vi "Calculation for heating four glasses.vi"(0 "Заданная температура":dbl[](array[numeric]), 1 "Текущая температура":dbl[](array[numeric]), 2 "Прошлая температура":dbl[](array[numeric]), 3 "Суммарная (прошлая) температура":dbl[](array[numeric]), 4 "Время прошлое":dbl[](array[numeric]), 5 "Время настоящее":dbl[](array[numeric])) -> (14 "Время во включенном состоянии":dbl[](array[numeric]), 19 "Суммарная температура":dbl[](array[numeric]))   [LabVIEW 2016]
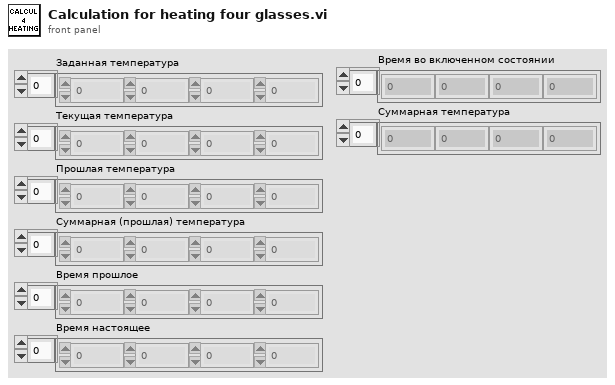
[diagram p1: front panel]
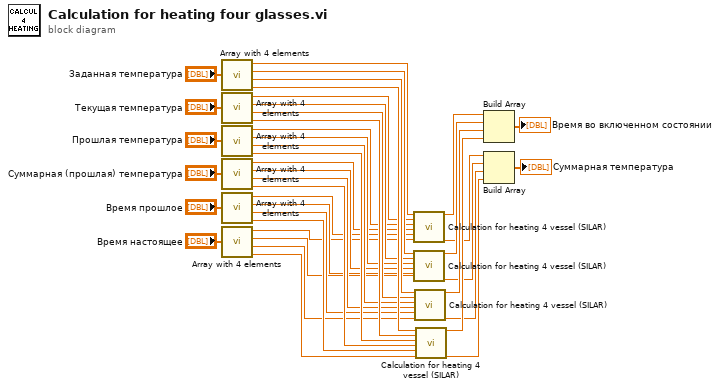
[diagram p0: block diagram]
diagram:
  n1 = call "Array with 4 elements.vi"("Array with 4 elements"="Заданная температура") -> ("element 3"=w35:dbl, "element 2"=w36:dbl, "element 1"=w38:dbl, "element 0"=w39:dbl)  [unwired: 7 in]
  n2 = call "Array with 4 elements.vi"("Array with 4 elements"="Текущая температура") -> ("element 3"=w31:dbl, "element 2"=w32:dbl, "element 1"=w33:dbl, "element 0"=w34:dbl)  [unwired: 7 in]
  n3 = call "Array with 4 elements.vi"("Array with 4 elements"="Прошлая температура") -> ("element 3"=w26:dbl, "element 2"=w27:dbl, "element 1"=w28:dbl, "element 0"=w29:dbl)  [unwired: 7 in]
  n4 = call "Array with 4 elements.vi"("Array with 4 elements"="Суммарная (прошлая) температура") -> ("element 3"=w21:dbl, "element 2"=w22:dbl, "element 1"=w23:dbl, "element 0"=w24:dbl)  [unwired: 7 in]
  n5 = call "Array with 4 elements.vi"("Array with 4 elements"="Время прошлое") -> ("element 3"=w16:dbl, "element 2"=w17:dbl, "element 1"=w18:dbl, "element 0"=w19:dbl)  [unwired: 7 in]
  n6 = call "Array with 4 elements.vi"("Array with 4 elements"="Время настоящее") -> ("element 3"=w11:dbl, "element 2"=w12:dbl, "element 1"=w13:dbl, "element 0"=w14:dbl)  [unwired: 7 in]
  n7 = call "Calculation for heating 4 vessel (SILAR).vi"("Tz - заданная температура"=w39, "Tt - текущая температура"=w34, "Ttp - текущая (прошлая) температура"=w29, "Tsp - суммарная (прошлая) температура"=w24, "tp - время прошлое"=w19, "tn - время настоящее"=w14) -> ("t1 - время во включенном состоянии"=w9:dbl, "Ts - суммарная температура"=w4:dbl)  [unwired: 12 in]
  n8 = call "Calculation for heating 4 vessel (SILAR).vi"("Tz - заданная температура"=w38, "Tt - текущая температура"=w33, "Ttp - текущая (прошлая) температура"=w28, "Tsp - суммарная (прошлая) температура"=w23, "tp - время прошлое"=w18, "tn - время настоящее"=w13) -> ("t1 - время во включенном состоянии"=w8:dbl, "Ts - суммарная температура"=w3:dbl)  [unwired: 12 in]
  n9 = call "Calculation for heating 4 vessel (SILAR).vi"("Tz - заданная температура"=w36, "Tt - текущая температура"=w32, "Ttp - текущая (прошлая) температура"=w27, "Tsp - суммарная (прошлая) температура"=w22, "tp - время прошлое"=w17, "tn - время настоящее"=w12) -> ("t1 - время во включенном состоянии"=w7:dbl, "Ts - суммарная температура"=w2:dbl)  [unwired: 12 in]
  n10 = call "Calculation for heating 4 vessel (SILAR).vi"("Tz - заданная температура"=w35, "Tt - текущая температура"=w31, "Ttp - текущая (прошлая) температура"=w26, "Tsp - суммарная (прошлая) температура"=w21, "tp - время прошлое"=w16, "tn - время настоящее"=w11) -> ("t1 - время во включенном состоянии"=w6:dbl, "Ts - суммарная температура"=w1:dbl)  [unwired: 12 in]
  n11 = Build Array(w9, w8, w7, w6) -> (→"Время во включенном состоянии":dbl[])
  n12 = Build Array(w4, w3, w2, w1) -> (→"Суммарная температура":dbl[])
